vi "DSF.Execution.Runtime.Plugin Manager.Load Plugin from Disk.vi"(8 "error in (no error)":errorcluster, 10 "path to Plugin":path, 11 "Plugin Manager in":refnum<class "Plugin Manager.lvclass">) -> (0 "error out":errorcluster, 2 "Plugin":refnum<class "DSF.Engine.Runtime.Plugin.lvclass">, 3 "Plugin Manager out":refnum<class "Plugin Manager.lvclass">)   [LabVIEW 2016, in "DSF.Engine.lvlib" / "Plugin Manager.lvclass"]
uses:
  Plugin Manager.lvclass
  Plugin/DSF.Engine.Runtime.Plugin.lvclass
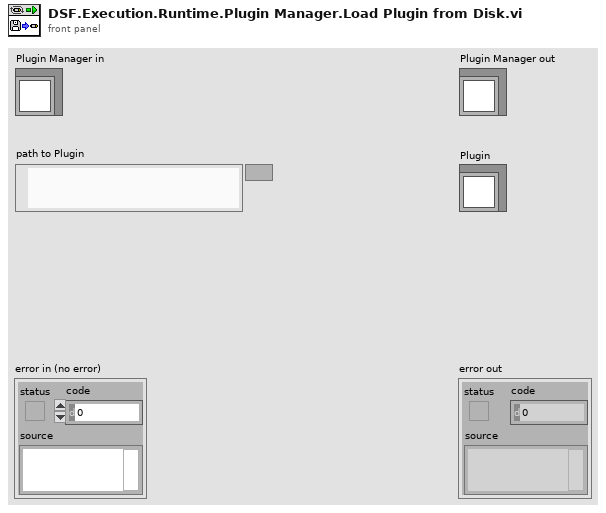
[diagram p1: front panel]
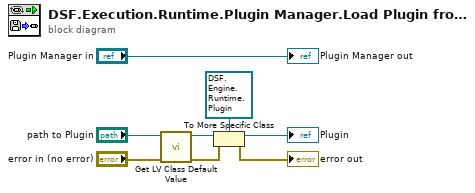
[diagram p0: block diagram]
diagram:
  n1 = call <vilib>:"Get LV Class Default Value.vi"("error in (no error)"="error in (no error)", "class path"="path to Plugin") -> ("error out"=w2:errorcluster, "object"=w5:refnum<class>)  [unwired: 8 in]
  n2 = To More Specific Class(target class=refnum<class "DSF.Engine.Runtime.Plugin.lvclass"> refnum ("Plugin"), reference=w5, error in=w2) -> (specific class reference=→"Plugin":refnum<class "DSF.Engine.Runtime.Plugin.lvclass">, error out=→"error out":errorcluster)
  "Plugin Manager out" <- "Plugin Manager in"
